vi "persist_controls_auto.vi"   [LabVIEW 2015]
uses:
  _persist_controls_polys.lvlib
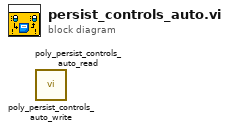
[diagram p0: block diagram]
diagram:
  n1 = call "poly_persist_controls_auto_write.vi"() -> ()  [unwired: 10 in, 2 out]
  n2 = call "poly_persist_controls_auto_read.vi"() -> ()  [unwired: 10 in, 2 out]
